vi "Queue Data log module.vi"(8 "error in":errorcluster) -> (0 "error out":errorcluster)   [LabVIEW 2020]
uses:
  Controls/Datalog enum.ctl
  Globals/Phase III Globals.vi
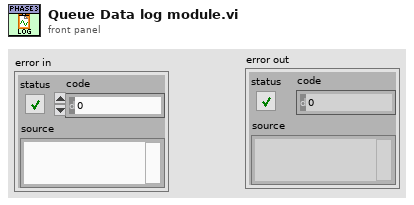
[diagram p1: front panel]
types:
  T1 = cluster{"Log In Progress?":bool, "Log Start Time":timestamp, "Analog Queues":refnum<queue>[], "Digital Queues":refnum<queue>[], "tdms file ref":refnum<k34>}
  T2 = typedef "Datalog enum.ctl" = enum16{"Initialize", "Poll", "Create file", "log Analog", "log Digital", "Flush Queues", "Close file", "Error", "Exit"}
  T3 = enum16{"open", "open or create", "create or replace", "create", "open (read-only)"}
  T4 = typedef "file folder ctl.ctl" = cluster{"Datalog path":path, "Configuration path":path, "Signal list path":path, "Sub vi's":path, "Authentication":path}
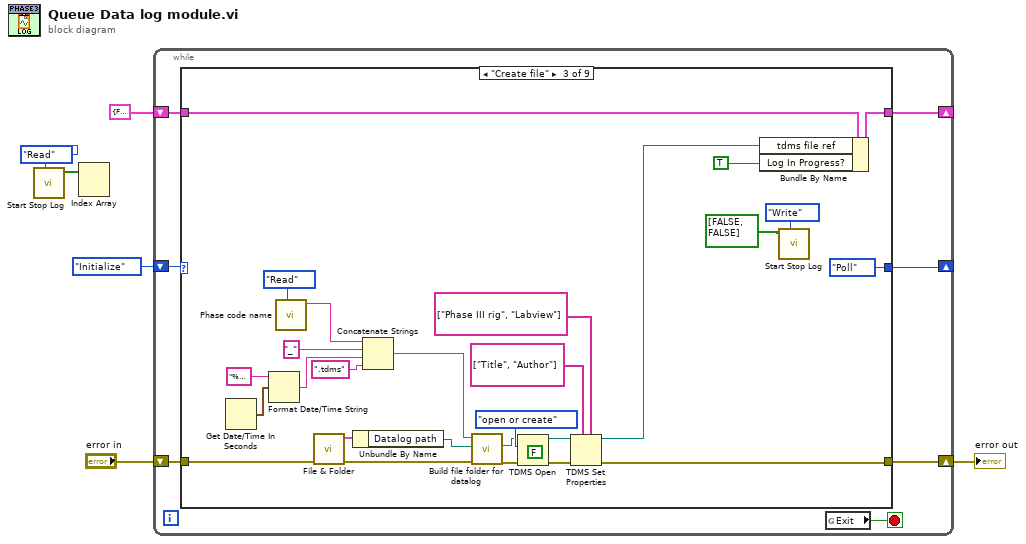
[diagram p0: block diagram]
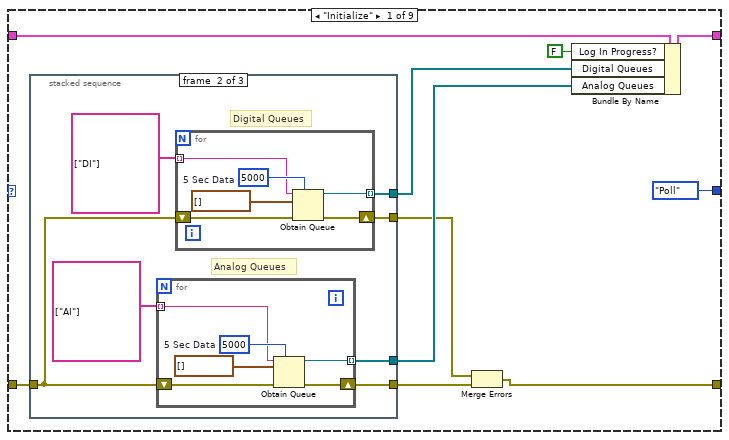
[diagram p2: hidden frame]
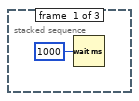
[diagram p3: hidden frame]
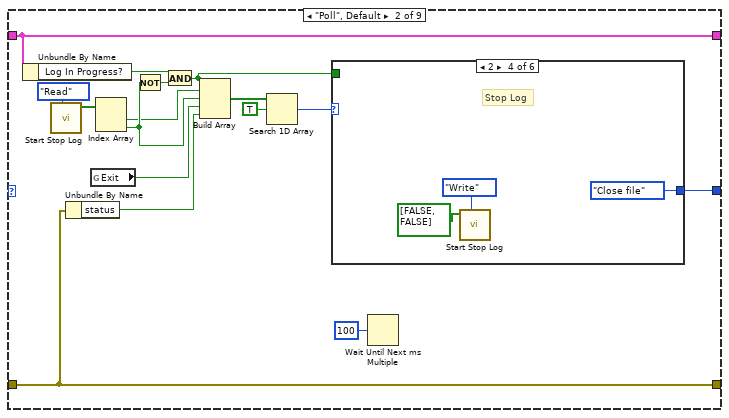
[diagram p5: hidden frame]
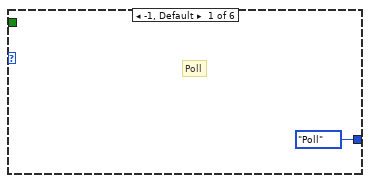
[diagram p6: hidden frame]
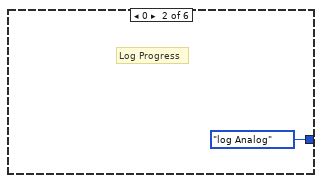
[diagram p7: hidden frame]
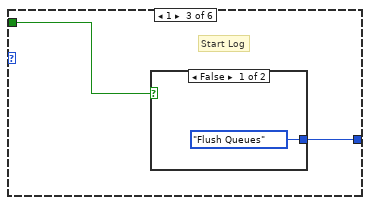
[diagram p8: hidden frame]
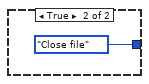
[diagram p9: hidden frame]
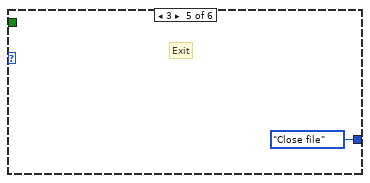
[diagram p10: hidden frame]
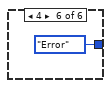
[diagram p11: hidden frame]
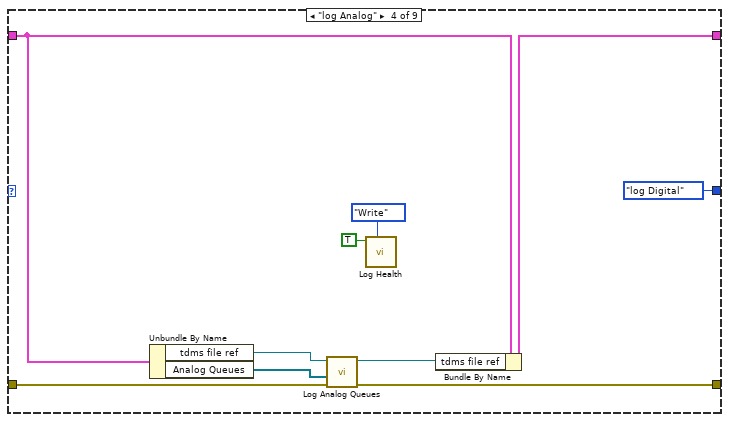
[diagram p12: hidden frame]
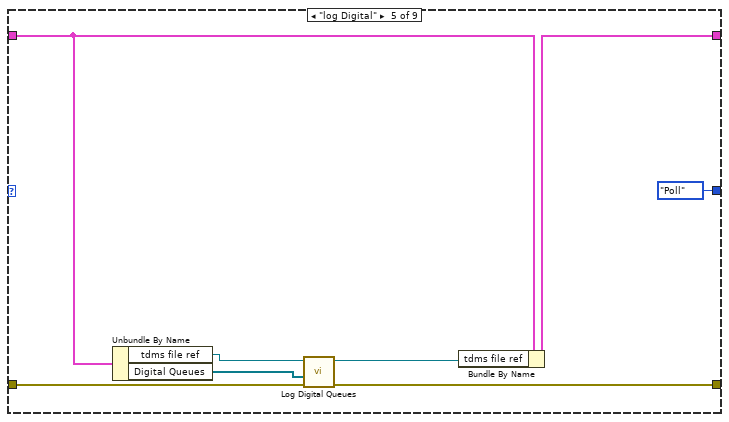
[diagram p13: hidden frame]
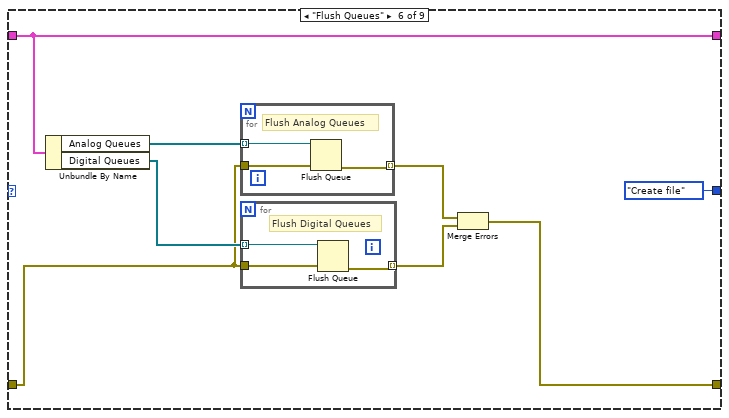
[diagram p14: hidden frame]
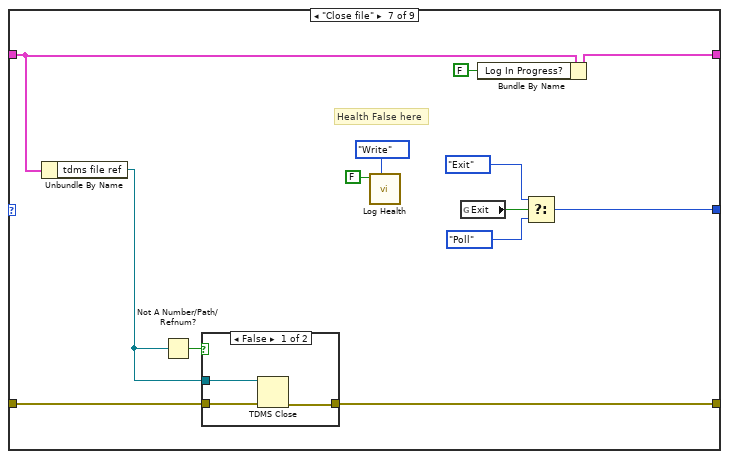
[diagram p15: hidden frame]
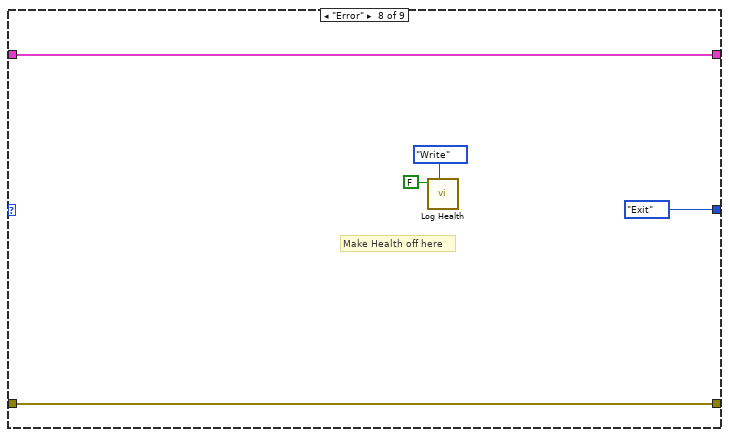
[diagram p17: hidden frame]
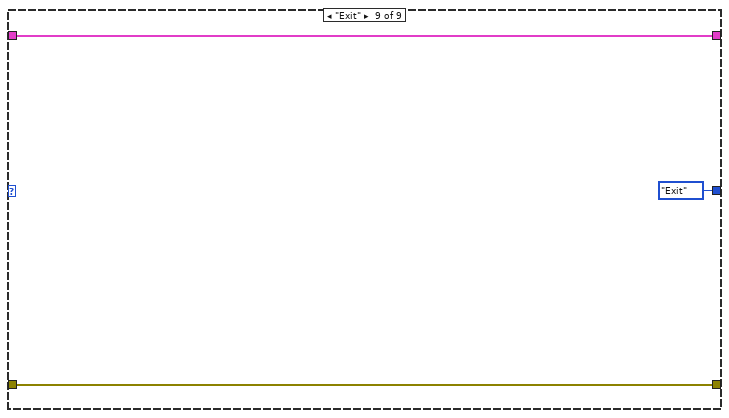
[diagram p18: hidden frame]
diagram:
  n1 = call "Start Stop Log.vi"("Enum"=enum16{"Read", "Write"}."Read") -> ("Start Stop log R"=w2:bool[])  [unwired: 9 in, 1 out]
  n2 = Index Array(array=w2) -> ()  [unwired: 2 in, 2 out]
  n3 = while {
    shift-right: [w8] -> _
    shift-left: Datalog_enum."Initialize" -> [w13]
    shift-right: [w10] -> _
    shift-left: T1 {"Log In Progress?"=FALSE, "Log Start Time"=timestamp(0 s since 1904-01-01), "Analog Queues"=[], "Digital Queues"=[], "tdms file ref"=refnum} -> [w11]
    shift-right: [w9] -> w3
    shift-left: "error in" -> [w12]
    stop <- w7 stop-if-true
    n4 = case shown="\"Create file\"" w13 {
      tunnel: w12 -> [w22 w53 w91 w104 w114 w119 w135 w149 w153]
      tunnel: w11 -> [w23 w59 w80 w106 w112 w122 w136 w151 w154]
      tunnel: [w21 w59 w79 w101 w109 w122 w139 w151 w154] -> w10
      tunnel: [w15 w53 w76 w103 w113 w116 w134 w149 w153] -> w9
      tunnel: [Datalog_enum."Poll" w54 Datalog_enum."Poll" Datalog_enum."log Digital" Datalog_enum."Poll" Datalog_enum."Create file" w140 Datalog_enum."Exit" Datalog_enum."Exit"] -> w8
      frame "Initialize" {
        n5 = stacked-sequence {
          tunnel: w22 -> [_ w28 _]
          tunnel: [_ w30 _] -> w18
          tunnel: [_ w27 _] -> w19
          tunnel: [_ w26 _] -> w17
          tunnel: [_ w25 _] -> w16
          frame #0 {
            n6 = Wait (ms)(milliseconds to wait=u32 1000) -> ()  [unwired: 1 out]
          }
          frame #1 {
            # "Digital Queues"
            # "Analog Queues"
            n7 = for {
              tunnel: [w40] -> w30 mode=indexing
              shift-right: [w42] -> w25
              shift-left: w28 -> [w43]
              tunnel: string[] ["AI"] -> [w39] mode=indexing
              w41 = 5000  # 5 Sec Data
              n8 = Obtain Queue(max queue size (-1, unlimited)=w41, name (unnamed)=w39, element data type=waveform(dbl)[] [] ("data"), error in (no error)=w43) -> (queue out=w40:refnum<queue>, error out=w42:errorcluster)  [unwired: 1 in, 1 out]
            }
            n9 = for {
              tunnel: [w34] -> w27 mode=indexing
              shift-right: [w36] -> w26
              shift-left: w28 -> [w37]
              tunnel: string[] ["DI"] -> [w33] mode=indexing
              w35 = 5000  # 5 Sec Data
              n10 = Obtain Queue(max queue size (-1, unlimited)=w35, name (unnamed)=w33, element data type=digitalwaveform[] [] ("data"), error in (no error)=w37) -> (queue out=w34:refnum<queue>, error out=w36:errorcluster)  [unwired: 1 in, 1 out]
            }
          }
          frame #2 {
            # "Datalog loop running Status"
          }
        }
        n11 = Merge Errors(w17, w16) -> (w15:errorcluster)
        n12 = Bundle By Name(cluster=w23, "Log In Progress?"=FALSE, "Digital Queues"=w19, "Analog Queues"=w18) -> (w21:T1)
      }
      frame "Poll", Default {
        n13 = Unbundle By Name(w59) -> ("Log In Progress?"=w50:bool)
        n14 = call "Start Stop Log.vi"("Enum"=enum16{"Read", "Write"}."Read") -> ("Start Stop log R"=w47:bool[])  [unwired: 9 in, 1 out]
        n15 = Unbundle By Name(w53) -> ("status"=w58:bool)
        n16 = global read "Phase III Globals.vi" "Exit"() -> (w52:bool)
        n17 = Index Array(array=w47) -> (element #1=w44:bool, element #2=w45:bool)  [unwired: 2 in]
        n18 = Not(x=w45) -> (.not. x?=w49:bool)
        n19 = And(x=w50, y=w49) -> (x .and. y?=w48:bool)
        n20 = Build Array(w48, w44, w45, w52, w58) -> (w57:bool[])
        n21 = Search 1D Array(1D array=w57, element=TRUE) -> (index of element=w55:i32)  [unwired: 1 in]
        n22 = case shown="2" w55 {
          tunnel: [Datalog_enum."Poll" Datalog_enum."log Analog" w63 Datalog_enum."Close file" Datalog_enum."Close file" Datalog_enum."Error"] -> w54
          tunnel: w48 -> [_ _ w62 _ _ _]
          frame -1, Default {
            # "Poll"
          }
          frame 0 {
            # "Log Progress"
          }
          frame 1 {
            # "Start Log"
            n23 = case shown="False" w62 {
              tunnel: [Datalog_enum."Flush Queues" Datalog_enum."Close file"] -> w63
              frame False {
              }
              frame True {
              }
            }
          }
          frame 2 {
            # "Stop Log"
            n24 = call "Start Stop Log.vi"("Enum"=enum16{"Read", "Write"}."Write", "Start Stop log"=bool[] [FALSE, FALSE]) -> ()  [unwired: 8 in, 2 out]
          }
          frame 3 {
            # "Exit"
          }
          frame 4 {
          }
        }
        n25 = Wait Until Next ms Multiple(millisecond multiple=u32 100) -> ()  [unwired: 1 out]
      }
      frame "Create file" {
        (unwired) FALSE ("disable buffering? (T)")
        n26 = Get Date/Time In Seconds() -> (seconds since 1Jan1904=w93:timestamp)
        n27 = Format Date/Time String(time format string (%c)="%Y_%b_%d_%Hh_%Mm_%Ssec", seconds (now)=w93) -> (date/time string=w97:string)  [unwired: 1 in]
        n28 = call "Phase code name.vi"("Enum"=enum16{"Read", "Write"}."Read") -> ("Phase codeR"=w73:string)  [unwired: 9 in, 1 out]
        n29 = call "File & Folder.vi"("error in (no error)"=w91) -> ("error out"=w90:errorcluster, "File Output"=w89:T4)  [unwired: 9 in]
        n30 = Unbundle By Name(w89) -> ("Datalog path"=w88:path)
        n31 = Concatenate Strings(w73, "_" ("string"), w97, ".tdms" ("string")) -> (w92:string)
        n32 = call "Build file folder for datalog.vi"("error in (no error)"=w90, "Base Path"=w88, "File Name"=w92) -> ("error out"=w82:errorcluster, "Result File path"=w81:path)  [unwired: 6 in, 1 out]
        n33 = TDMS Open(8:w82, 10:T3."open or create" ("operation (0:open)"), 11:w81) -> (0:w86:errorcluster, 3:w85:refnum<k34>)  [unwired: 4 in]
        n34 = TDMS Set Properties(5:string[] ["Phase III rig", "Labview"] ("property names"), 7:string[] ["Title", "Author"] ("property names"), 8:w86, 11:w85) -> (0:w76:errorcluster, 3:w78:refnum<k34>)  [unwired: 4 out]
        n35 = Bundle By Name(cluster=w80, "tdms file ref"=w78, "Log In Progress?"=TRUE) -> (w79:T1)
        n36 = call "Start Stop Log.vi"("Enum"=enum16{"Read", "Write"}."Write", "Start Stop log"=bool[] [FALSE, FALSE]) -> ()  [unwired: 8 in, 2 out]
      }
      frame "log Analog" {
        n37 = Unbundle By Name(w106) -> ("tdms file ref"=w102:refnum<k34>, "Analog Queues"=w105:refnum<queue>[])
        n38 = call "Log Analog Queues.vi"("error in"=w104, "Analog queues"=w105, "tdms file in"=w102) -> ("error out"=w103:errorcluster, "tdms ref out"=w100:refnum<k34>)  [unwired: 7 in]
        n39 = call "Log Health.vi"("Enum"=enum16{"Read", "Write"}."Write", "Log health"=TRUE) -> ()  [unwired: 8 in, 2 out]
        n40 = Bundle By Name(cluster=w106, "tdms file ref"=w100) -> (w101:T1)
      }
      frame "log Digital" {
        n41 = Unbundle By Name(w112) -> ("tdms file ref"=w111:refnum<k34>, "Digital Queues"=w110:refnum<queue>[])
        n42 = call "Log Digital Queues.vi"("error in"=w114, "DI_queue"=w110, "tdms file in"=w111) -> ("error out"=w113:errorcluster, "tdms file out"=w108:refnum<k34>)  [unwired: 7 in]
        n43 = Bundle By Name(cluster=w112, "tdms file ref"=w108) -> (w109:T1)
      }
      frame "Flush Queues" {
        n44 = Unbundle By Name(w122) -> ("Analog Queues"=w121:refnum<queue>[], "Digital Queues"=w120:refnum<queue>[])
        n45 = for {
          tunnel: w121 -> [w129] mode=indexing
          tunnel: w119 -> [w128]
          tunnel: [w127] -> w118 mode=indexing
          # "Flush Analog Queues"
          n46 = Flush Queue(queue=w129, error in (no error)=w128) -> (error out=w127:errorcluster)  [unwired: 2 out]
        }
        n47 = for {
          tunnel: w120 -> [w126] mode=indexing
          tunnel: w119 -> [w125]
          tunnel: [w124] -> w117 mode=indexing
          # "Flush Digital Queues"
          n48 = Flush Queue(queue=w126, error in (no error)=w125) -> (error out=w124:errorcluster)  [unwired: 2 out]
        }
        n49 = Merge Errors(w118, w117) -> (w116:errorcluster)
      }
      frame "Close file" {
        # "Health False here"
        n50 = Unbundle By Name(w136) -> ("tdms file ref"=w132:refnum<k34>)
        n51 = Not A Number/Path/Refnum?(number/path/refnum=w132) -> (NaN/Path/Refnum?=w133:bool)
        n52 = case shown="False" w133 {
          tunnel: w135 -> [w145 w146]
          tunnel: [w144 w146] -> w134
          tunnel: w132 -> [w143 _]
          frame False {
            n53 = TDMS Close(8:w145, 11:w143) -> (0:w144:errorcluster)  [unwired: 1 out]
          }
          frame True {
          }
        }
        n54 = call "Log Health.vi"("Enum"=enum16{"Read", "Write"}."Write", "Log health"=FALSE) -> ()  [unwired: 8 in, 2 out]
        n55 = global read "Phase III Globals.vi" "Exit"() -> (w137:bool)
        n56 = Bundle By Name(cluster=w136, "Log In Progress?"=FALSE) -> (w139:T1)
        n57 = Select(t=Datalog_enum."Exit", s=w137, f=Datalog_enum."Poll") -> (s? t:f=w140:T2)
      }
      frame "Error" {
        # "Make Health off here"
        n58 = call "Log Health.vi"("Enum"=enum16{"Read", "Write"}."Write", "Log health"=FALSE) -> ()  [unwired: 8 in, 2 out]
      }
      frame "Exit" {
      }
    }
    n59 = global read "Phase III Globals.vi" "Exit"() -> (w7:bool)
  }
  "error out" <- w3
